vi "storeADCMixedToArray-wang-test2.vi"(0 "String":string) -> (14 "dataADCArray 2":i32[](array[numeric]), 18 "Graph Data":T1)   [LabVIEW 2014]
uses:
  testproj/controls/Graph Data.ctl
  <vilib>/Utility/miscctls.llb/LVAnnotationListTypeDef.ctl
  <vilib>/Utility/miscctls.llb/LVCursorListTypeDef.ctl
panel:
  out "Waveform":waveform(dbl)
  out "Graph":waveform(i32)[](graph)
  out "channel 2":u8[](array[numeric])
  out "Numeric 2":dbl
  out "Numeric":i32
  out "CH7":i32[](array[numeric])
  out "CH6":i32[](array[numeric])
  out "CH5":i32[](array[numeric])
  out "CH4":i32[](array[numeric])
  out "CH3":i32[](array[numeric])
  out "CH2":i32[](array[numeric])
  out "CH1":i32[](array[numeric])
  out "CH0":i32[](array[numeric])
  out "TotalTrigger":i32
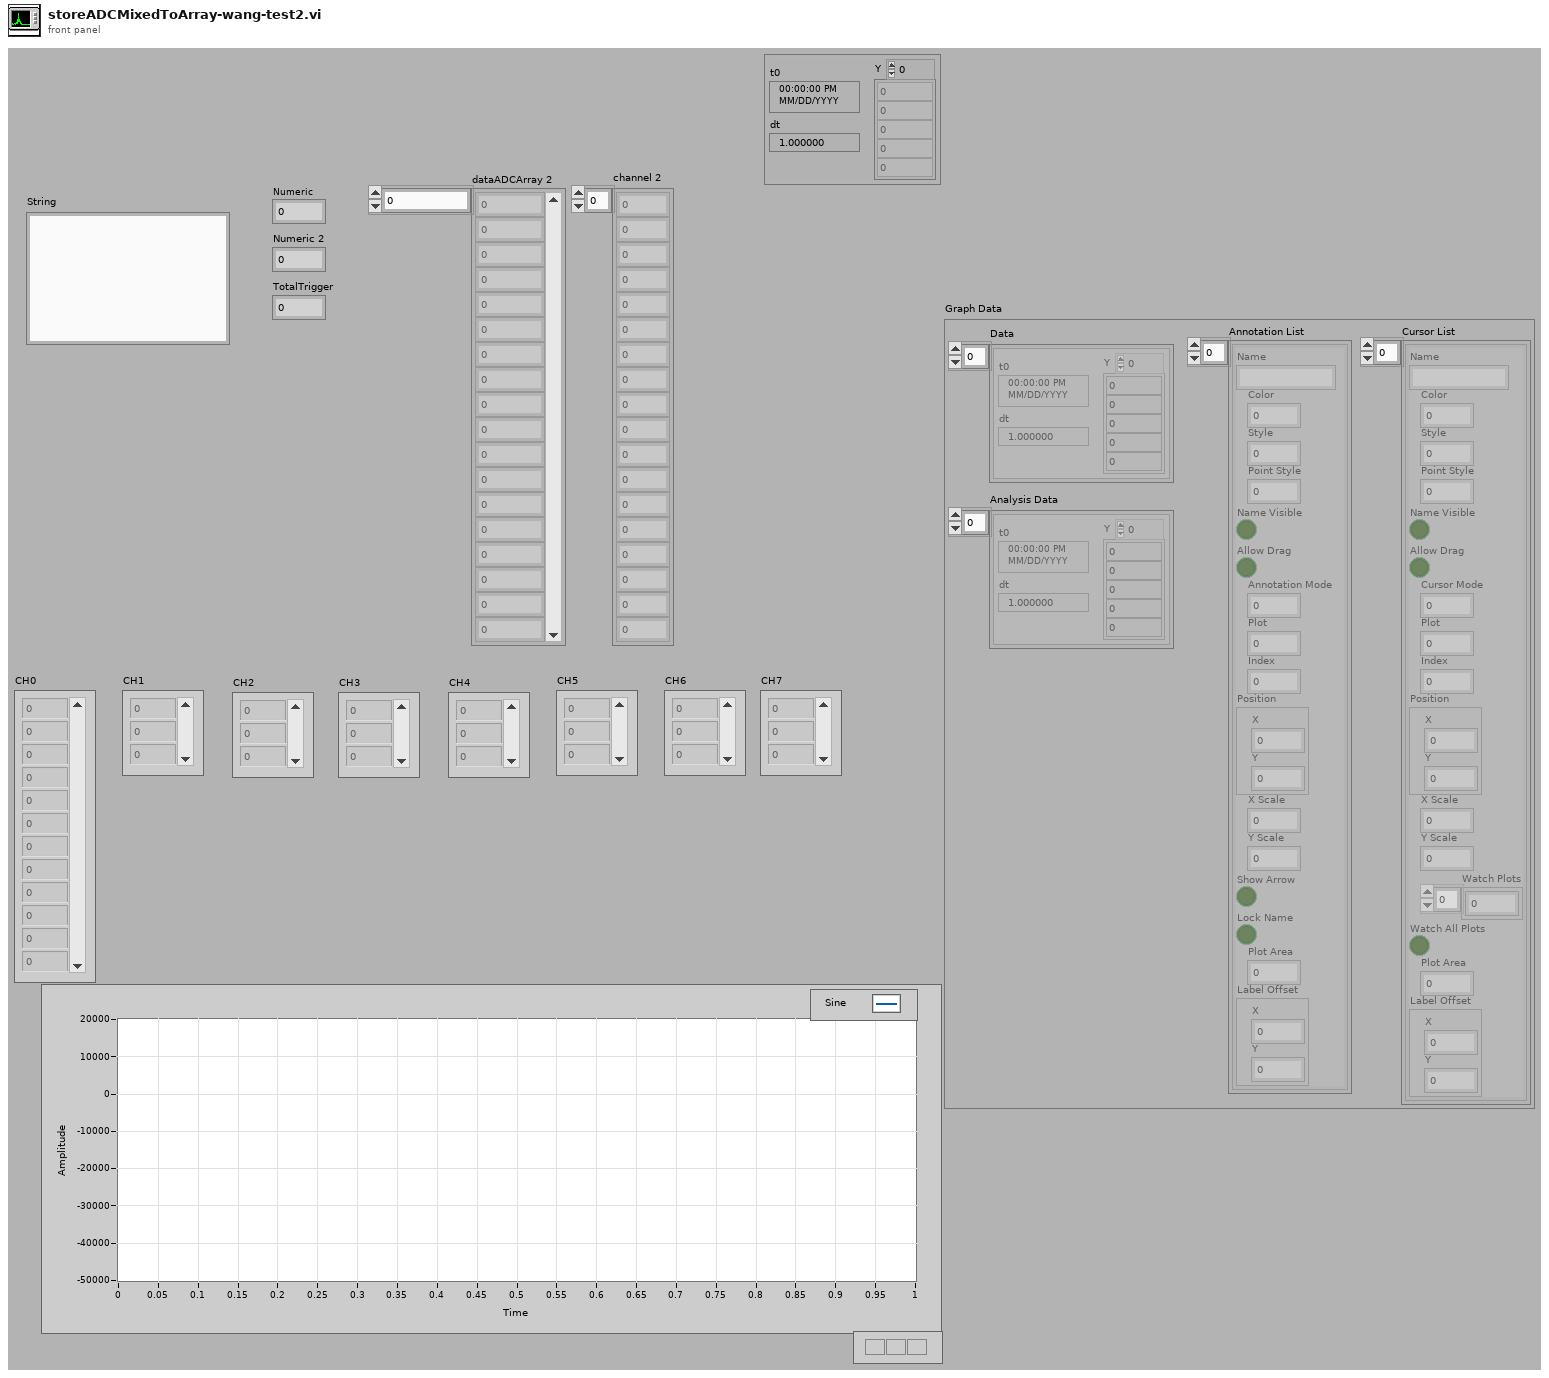
[diagram p1: front panel]
types:
  T1 = typedef "Graph Data.ctl" = cluster{"Data":waveform(dbl)[], "Annotation List":T2, "Cursor List":T3, "Analysis Data":waveform(dbl)[]}
  T2 = typedef "LVAnnotationListTypeDef.ctl" = cluster{"Name":string, "Color":u32, "Style":u8, "Point Style":u8, "Name Visible":bool, "Allow Drag":bool, "Annotation Mode":u32, "Plot":i32, "Index":i32, "Position":cluster{"X":dbl, "Y":dbl}, "X Scale":u32, "Y Scale":u32, "Show Arrow":bool, "Lock Name":bool, "Plot Area":i32, "Label Offset":cluster{"X":dbl, "Y":dbl}}[]
  T3 = typedef "LVCursorListTypeDef.ctl" = cluster{"Name":string, "Color":u32, "Style":u8, "Point Style":u8, "Name Visible":bool, "Allow Drag":bool, "Cursor Mode":u32, "Plot":i32, "Index":i32, "Position":cluster{"X":dbl, "Y":dbl}, "X Scale":u32, "Y Scale":u32, "Watch Plots":i32[], "Watch All Plots":bool, "Plot Area":i32, "Label Offset":cluster{"X":dbl, "Y":dbl}}[]
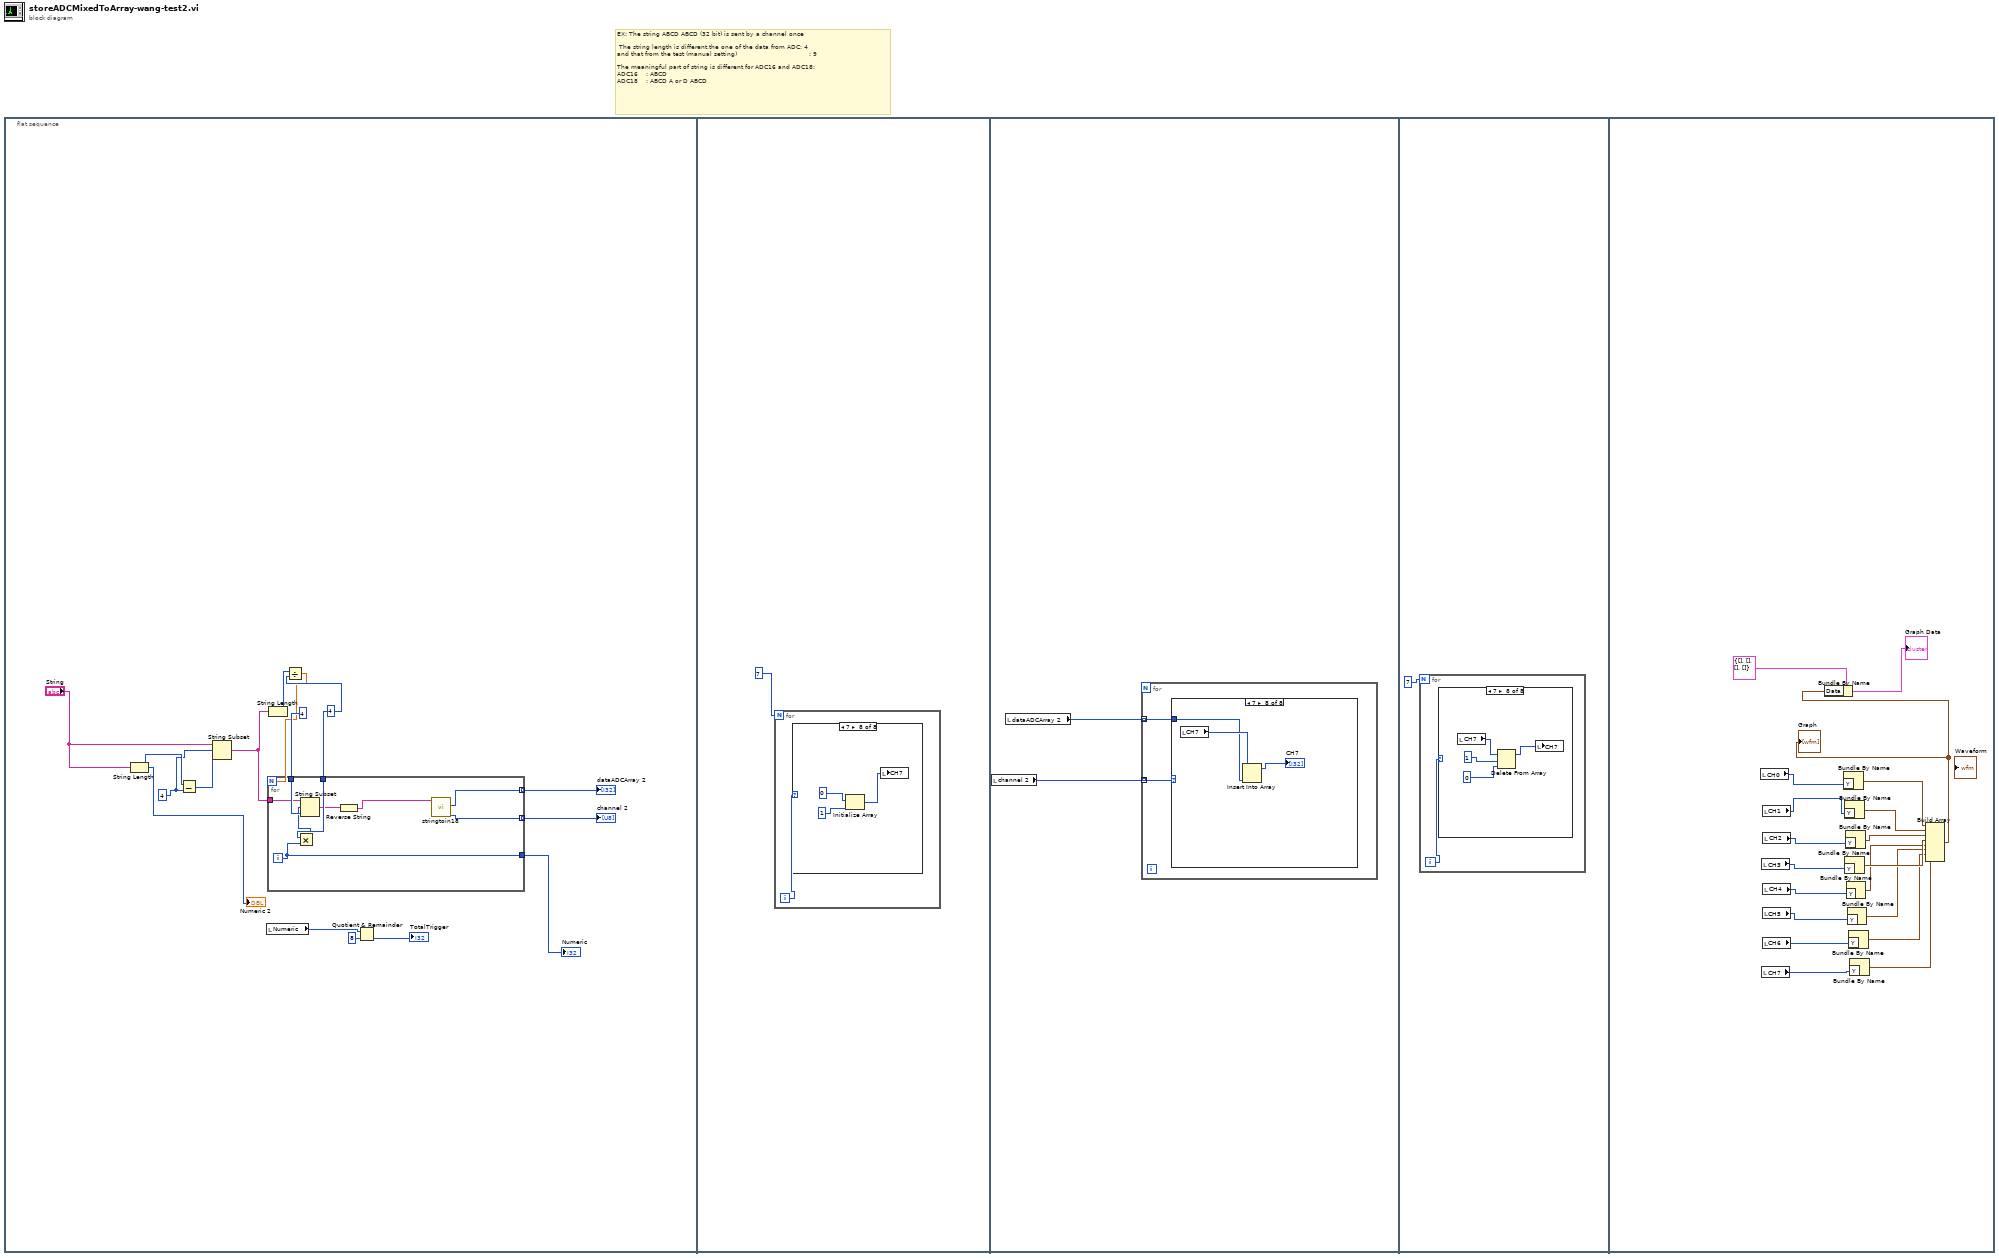
[diagram p0: block diagram]
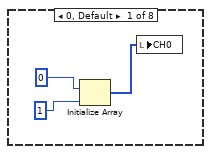
[diagram p2: hidden frame]
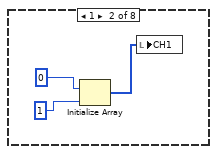
[diagram p3: hidden frame]
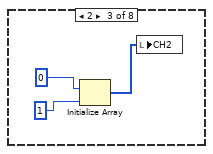
[diagram p4: hidden frame]
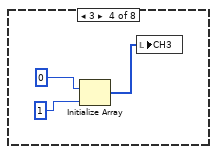
[diagram p5: hidden frame]
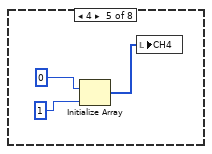
[diagram p6: hidden frame]
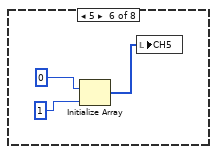
[diagram p7: hidden frame]
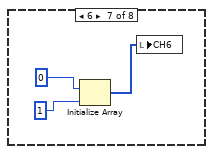
[diagram p8: hidden frame]
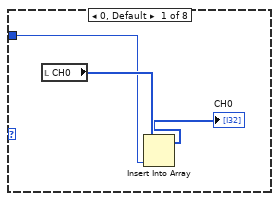
[diagram p9: hidden frame]
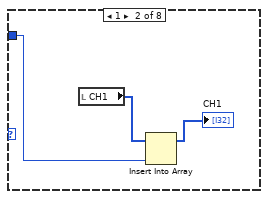
[diagram p10: hidden frame]
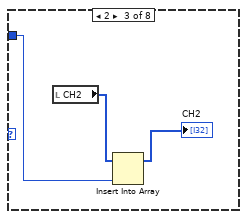
[diagram p11: hidden frame]
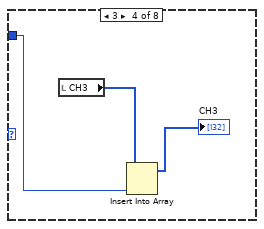
[diagram p12: hidden frame]
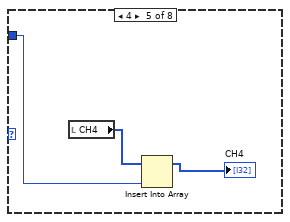
[diagram p13: hidden frame]
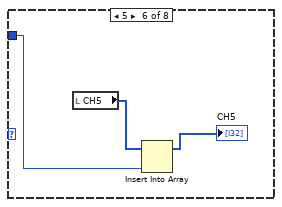
[diagram p14: hidden frame]
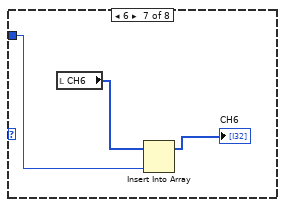
[diagram p15: hidden frame]
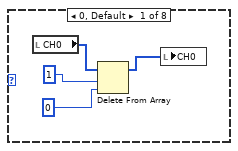
[diagram p16: hidden frame]
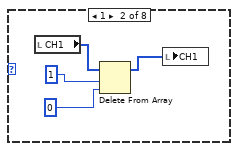
[diagram p17: hidden frame]
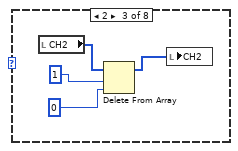
[diagram p18: hidden frame]
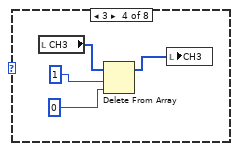
[diagram p19: hidden frame]
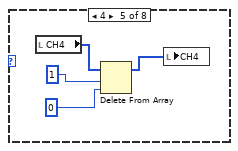
[diagram p20: hidden frame]
diagram:
  # "EX: The string ABCD ABCD (32 bit) is sent by a channel once                \n\n The string length is different,the one of the data from ADC: 4\nand that from the test (manual setting)                                    : 9\n\nThe meaningful part of string is different for ADC16 and ADC18:\nADC16    : ABCD                          \nADC18    : ABCD A or D ABCD"
  n1 = flat-sequence {
    frame #0 {
      w9 = 4
      w12 = 4
      n2 = String Length(string="String") -> (length=w15:i32)
      "Numeric 2" <- w15
      n3 = Subtract(x=w15, y=w12) -> (x-y=w13:i32)
      n4 = String Subset(string="String", offset (0)=w12, length (rest)=w13) -> (substring=w6:string)
      n5 = local read "Numeric"() -> (w3:i32)
      n6 = String Length(string=w6) -> (length=w10:i32)
      n7 = Divide(x=w10, y=w9) -> (x/y=w8:dbl)
      n8 = for {
        N: w8 -> [_]
        tunnel: 4 -> [w24]
        tunnel: w9 -> [w23]
        tunnel: [w19] -> w14
        tunnel: w6 -> [w20]
        tunnel: [w17] -> w2 mode=indexing
        tunnel: [w16] -> w1 mode=indexing
        i -> [w19]
        n9 = Multiply(x=w23, y=w19) -> (x*y=w22:i32)
        n10 = String Subset(string=w20, offset (0)=w22, length (rest)=w24) -> (substring=w21:string)
        n11 = Reverse String(1:w21) -> (0:w18:string)
        n12 = call "stringtoin18.vi"("input_string"=w18) -> ("channel"=w16:u8, "outputComplemented_int"=w17:i32)  [unwired: 7 in, 2 out]
      }
      "Numeric" <- w14
      "dataADCArray 2" <- w2
      "channel 2" <- w1
      n13 = Quotient & Remainder(x=w3, y=8) -> (floor(x/y)=→"TotalTrigger":i32)  [unwired: 1 out]
    }
    frame #1 {
      n14 = for {
        N: 7 -> [_]
        i -> [w26]
        n15 = case shown="7" w26 {
          frame 0, Default {
            n16 = Initialize Array(0, 1) -> (w27:i32[])
            n17 = local write "CH0"(w27) -> ()
          }
          frame 1 {
            n18 = Initialize Array(0, 1) -> (w30:i32[])
            n19 = local write "CH1"(w30) -> ()
          }
          frame 2 {
            n20 = Initialize Array(0, 1) -> (w33:i32[])
            n21 = local write "CH2"(w33) -> ()
          }
          frame 3 {
            n22 = Initialize Array(0, 1) -> (w36:i32[])
            n23 = local write "CH3"(w36) -> ()
          }
          frame 4 {
            n24 = Initialize Array(0, 1) -> (w39:i32[])
            n25 = local write "CH4"(w39) -> ()
          }
          frame 5 {
            n26 = Initialize Array(0, 1) -> (w42:i32[])
            n27 = local write "CH5"(w42) -> ()
          }
          frame 6 {
            n28 = Initialize Array(0, 1) -> (w45:i32[])
            n29 = local write "CH6"(w45) -> ()
          }
          frame 7 {
            n30 = Initialize Array(0, 1) -> (w48:i32[])
            n31 = local write "CH7"(w48) -> ()
          }
        }
      }
    }
    frame #2 {
      n32 = local read "channel 2"() -> (w52:u8[])
      n33 = local read "dataADCArray 2"() -> (w51:i32[])
      n34 = for {
        tunnel: w52 -> [w54] mode=indexing
        tunnel: w51 -> [w53] mode=indexing
        n35 = case shown="7" w54 {
          tunnel: w53 -> [w55 w58 w61 w64 w67 w70 w73 w76]
          frame 0, Default {
            n36 = local read "CH0"() -> (w57:i32[])
            n37 = Insert Into Array(array=w57, new element=w55) -> (→"CH0":i32[])  [unwired: 1 in]
          }
          frame 1 {
            n38 = local read "CH1"() -> (w60:i32[])
            n39 = Insert Into Array(array=w60, new element=w58) -> (→"CH1":i32[])  [unwired: 1 in]
          }
          frame 2 {
            n40 = local read "CH2"() -> (w63:i32[])
            n41 = Insert Into Array(array=w63, new element=w61) -> (→"CH2":i32[])  [unwired: 1 in]
          }
          frame 3 {
            n42 = local read "CH3"() -> (w66:i32[])
            n43 = Insert Into Array(array=w66, new element=w64) -> (→"CH3":i32[])  [unwired: 1 in]
          }
          frame 4 {
            n44 = local read "CH4"() -> (w69:i32[])
            n45 = Insert Into Array(array=w69, new element=w67) -> (→"CH4":i32[])  [unwired: 1 in]
          }
          frame 5 {
            n46 = local read "CH5"() -> (w72:i32[])
            n47 = Insert Into Array(array=w72, new element=w70) -> (→"CH5":i32[])  [unwired: 1 in]
          }
          frame 6 {
            n48 = local read "CH6"() -> (w75:i32[])
            n49 = Insert Into Array(array=w75, new element=w73) -> (→"CH6":i32[])  [unwired: 1 in]
          }
          frame 7 {
            n50 = local read "CH7"() -> (w77:i32[])
            n51 = Insert Into Array(array=w77, new element=w76) -> (→"CH7":i32[])  [unwired: 1 in]
          }
        }
      }
    }
    frame #3 {
      n52 = for {
        N: 7 -> [_]
        i -> [w80]
        n53 = case shown="7" w80 {
          frame 0, Default {
            n54 = local read "CH0"() -> (w84:i32[])
            n55 = Delete From Array(array=w84, length=1, index=0) -> (array with subset deleted=w81:i32[])  [unwired: 1 out]
            n56 = local write "CH0"(w81) -> ()
          }
          frame 1 {
            n57 = local read "CH1"() -> (w88:i32[])
            n58 = Delete From Array(array=w88, length=1, index=0) -> (array with subset deleted=w85:i32[])  [unwired: 1 out]
            n59 = local write "CH1"(w85) -> ()
          }
          frame 2 {
            n60 = local read "CH2"() -> (w92:i32[])
            n61 = Delete From Array(array=w92, length=1, index=0) -> (array with subset deleted=w89:i32[])  [unwired: 1 out]
            n62 = local write "CH2"(w89) -> ()
          }
          frame 3 {
            n63 = local read "CH3"() -> (w96:i32[])
            n64 = Delete From Array(array=w96, length=1, index=0) -> (array with subset deleted=w93:i32[])  [unwired: 1 out]
            n65 = local write "CH3"(w93) -> ()
          }
          frame 4 {
            n66 = local read "CH4"() -> (w100:i32[])
            n67 = Delete From Array(array=w100, length=1, index=0) -> (array with subset deleted=w97:i32[])  [unwired: 1 out]
            n68 = local write "CH4"(w97) -> ()
          }
          frame 5 {
            n69 = local read "CH5"() -> (w104:i32[])
            n70 = Delete From Array(array=w104, length=1, index=0) -> (array with subset deleted=w101:i32[])  [unwired: 1 out]
            n71 = local write "CH5"(w101) -> ()
          }
          frame 6 {
            n72 = local read "CH6"() -> (w108:i32[])
            n73 = Delete From Array(array=w108, length=1, index=0) -> (array with subset deleted=w105:i32[])  [unwired: 1 out]
            n74 = local write "CH6"(w105) -> ()
          }
          frame 7 {
            n75 = local read "CH7"() -> (w112:i32[])
            n76 = Delete From Array(array=w112, length=1, index=0) -> (array with subset deleted=w109:i32[])  [unwired: 1 out]
            n77 = local write "CH7"(w109) -> ()
          }
        }
      }
    }
    frame #4 {
      n78 = local read "CH0"() -> (w131:i32[])
      n79 = local read "CH3"() -> (w123:i32[])
      n80 = local read "CH7"() -> (w127:i32[])
      n81 = local read "CH1"() -> (w129:i32[])
      n82 = local read "CH5"() -> (w125:i32[])
      n83 = local read "CH6"() -> (w126:i32[])
      n84 = local read "CH2"() -> (w122:i32[])
      n85 = local read "CH4"() -> (w124:i32[])
      n86 = Bundle By Name("Y"=w131) -> (w130:waveform(i32))  [unwired: 1 in]
      n87 = Bundle By Name("Y"=w129) -> (w128:waveform(i32))  [unwired: 1 in]
      n88 = Bundle By Name("Y"=w123) -> (w120:waveform(i32))  [unwired: 1 in]
      n89 = Bundle By Name("Y"=w122) -> (w121:waveform(i32))  [unwired: 1 in]
      n90 = Bundle By Name("Y"=w124) -> (w116:waveform(i32))  [unwired: 1 in]
      n91 = Bundle By Name("Y"=w125) -> (w119:waveform(i32))  [unwired: 1 in]
      n92 = Bundle By Name("Y"=w126) -> (w118:waveform(i32))  [unwired: 1 in]
      n93 = Bundle By Name("Y"=w127) -> (w117:waveform(i32))  [unwired: 1 in]
      n94 = Build Array(w130, w128, w121, w120, w116, w119, w118, w117) -> (w115:waveform(i32)[])
      "Graph" <- w115
      n95 = Bundle By Name(cluster=T1 {"Data"=[], "Annotation List"=[], "Cursor List"=[], "Analysis Data"=[]} ("Graph Data"), "Data"=w115) -> (→"Graph Data":T1)
    }
  }
